vi "SetParent.vi"(8 "error in (no error)":errorcluster, 10 "hWndParent (NULL)":T1, 11 "hWndChild (NULL)":T1) -> (0 "error out":errorcluster, 2 "hWndOldParent":T1, 3 "dup hWndChild":T1)   [LabVIEW 2011]
doc: "SetParent\nThe SetParent function changes the parent window of the specified child window. \n\nHWND SetParent(\n HWND hWndChild, // handle to window whose parent is changing\n HWND hWndNewParent // handle to new parent window\n);\n \nParameters\nhWndChild \nHandle to the child window. \nhWndNewParent \nHandle to the new parent window. If this parameter is NULL, the desktop window becomes the new parent window. \nWindows NT 5.0 and later: If this parameter is HWND_MESSAGE, the child window becomes a message-only window. \n\nReturn Values\nIf the function succeeds, the return value is a handle to the previous parent window.\n\nIf the function fails, the return value is NULL. To get extended error information, callGetLastError. \n\nRemarks\nAn application can use the SetParent function to set the parent window of a pop-up, overlapped, or child window. The new parent window and the child window must belong to the same application. \n\nIf the window identified by the hWndChild parameter is visible, the system performs the appropriate redrawing and repainting. \n\nFor compatibility reasons, SetParent does not modify the WS_CHILD or WS_POPUP window styles of the window whose parent is being changed. Therefore, if hWndNewParent is NULL, you should also clear the WS_CHILD bit and set the WS_POPUP style after calling SetParent. Conversely, if hWndNewParent is not NULL and the window was previously a child of the desktop, you should clear the WS_POPUP style and set the WS_CHILD style before calling SetParent."
uses:
  hWnd.ctl
  user32.dll
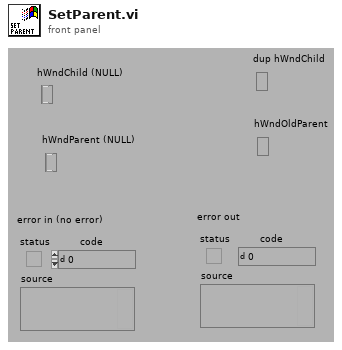
[diagram p1: front panel]
types:
  T1 = typedef "hWnd.ctl" = refnum<k1>
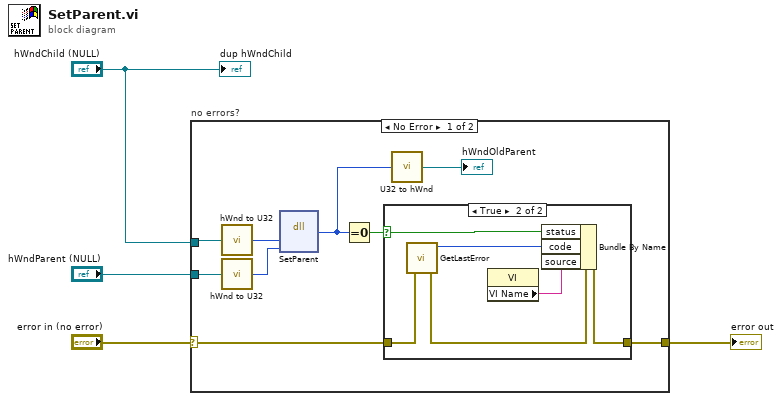
[diagram p0: block diagram]
diagram:
  n1 = case "no errors?" shown="No Error" "error in (no error)" {
    selector: "error in (no error)" -> [w10 w21]
    tunnel: [w11 w21] -> w4
    tunnel: "hWndParent (NULL)" -> [w8 _]
    tunnel: "hWndChild (NULL)" -> [w13 _]
    frame No Error {
      n2 = call "hWnd to U32.vi"("hWnd"=w13) -> ("hWnd"=w12:u32)  [unwired: 4 out]
      n3 = call "hWnd to U32.vi"("hWnd"=w8) -> ("hWnd"=w7:u32)  [unwired: 4 out]
      n4 = dll-call lib="user32.dll" fn="SetParent"("hWndChild"=w12, "hWndNewParent"=w7) -> ("hWndOldParent"=w6:u32)  [unwired: 5 in, 2 out]
      n5 = Equal To 0?(x=w6) -> (x = 0?=w9:bool)
      n6 = case shown="True" w9 {
        selector: w9 -> [_ w15]
        tunnel: w10 -> [w14 w19]
        tunnel: [w14 w20] -> w11
        frame False {
        }
        frame True {
          n7 = call "GetLastError.vi"("error in (no error)"=w19) -> ("error out"=w18:errorcluster, "CODE"=w17:i32)  [unwired: 5 out]
          n8 = property class="VI"() -> ("VI Name"=w16:string)  [unwired: 2 in, 2 out]
          n9 = Bundle By Name(cluster=w18, "status"=w15, "code"=w17, "source"=w16) -> (w20:errorcluster)
        }
      }
      n10 = call "U32 to hWnd.vi"("hWnd"=w6) -> ("hWnd"=→"hWndOldParent":T1)  [unwired: 4 out]
    }
    frame Error {
    }
  }
  "error out" <- w4
  "dup hWndChild" <- "hWndChild (NULL)"
